vi "format_data_ITM10.vi"(8 "value_array":dbl[](array[numeric]), 11 "time":timestamp) -> (3 "waveform_array":waveform(dbl)[](array[waveform]))   [LabVIEW 2019]
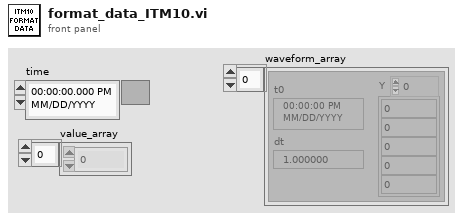
[diagram p1: front panel]
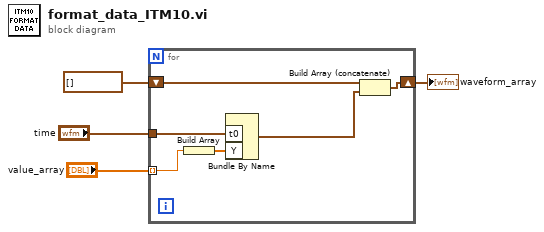
[diagram p0: block diagram]
diagram:
  n1 = for {
    tunnel: "time" -> [w9]
    tunnel: "value_array" -> [w8] mode=indexing
    shift-right: [w6] -> w1
    shift-left: waveform(dbl)[] [] -> [w5]
    n2 = Build Array(w8) -> (w10:dbl[])
    n3 = Bundle By Name("t0"=w9, "Y"=w10) -> (w7:waveform(dbl))  [unwired: 1 in]
    n4 = Build Array (concatenate)(w5, w7) -> (w6:waveform(dbl)[])
  }
  "waveform_array" <- w1
